vi "HW send config response.vi"(8 "error in (no error)":errorcluster, 10 "UE resp":refnum<class "UE_slave.lvclass">, 11 "mmWave instrument in":refnum<class "mmWave instrument.lvclass">) -> (0 "error out":errorcluster)   [LabVIEW 2019, in "HW Control.lvlib"]
uses:
  HW Control.lvlib
  SubVIs/mmWave instrument_class/mmWave instrument.lvclass
  Intertarget communication/UE_slave_class/UE_slave.lvclass
  SubVIs/Shared/System GV.vi
  SubVIs/Shared/Shared.lvlib
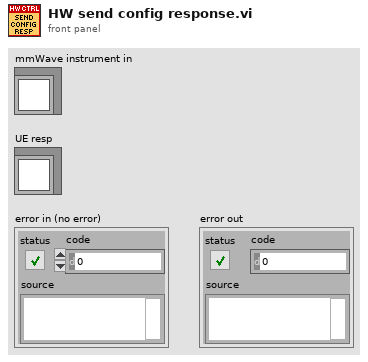
[diagram p1: front panel]
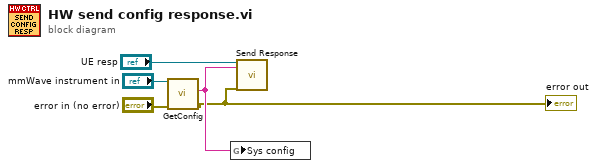
[diagram p0: block diagram]
diagram:
  n1 = call-dynamic "GetConfig.vi"("error in (no error)"="error in (no error)", "reference in"="mmWave instrument in") -> ("error out"=w4:errorcluster, "String"=w5:string)  [unwired: 7 in, 1 out]
  "error out" <- w4
  n2 = global write "System GV.vi" "Sys config"(w5) -> ()
  n3 = call-dynamic "Send Response.vi"("reference in"="UE resp", "response"=w5, "error in (no error)"=w4) -> ()  [unwired: 15 in, 2 out]
